vi "GCliWrite.vi"(8 "error in (no error)":errorcluster, 10 "Text to Write":string, 11 "CLI in":refnum<class "CLI.lvclass">) -> (0 "error out":errorcluster, 3 "CLI out":refnum<class "CLI.lvclass">)   [LabVIEW 2023, in "Reusables.lvlib"]
uses:
  Reusables.lvlib
  <vilib>/Wiresmith Technology/G CLI/CLI Class/CLI.lvclass
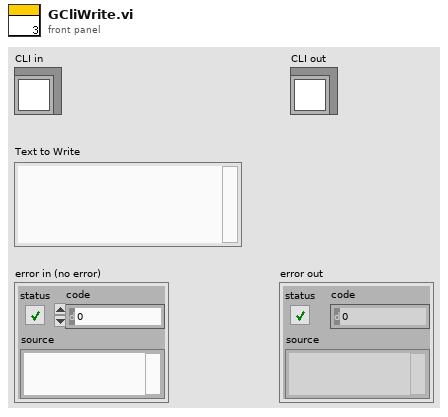
[diagram p1: front panel]
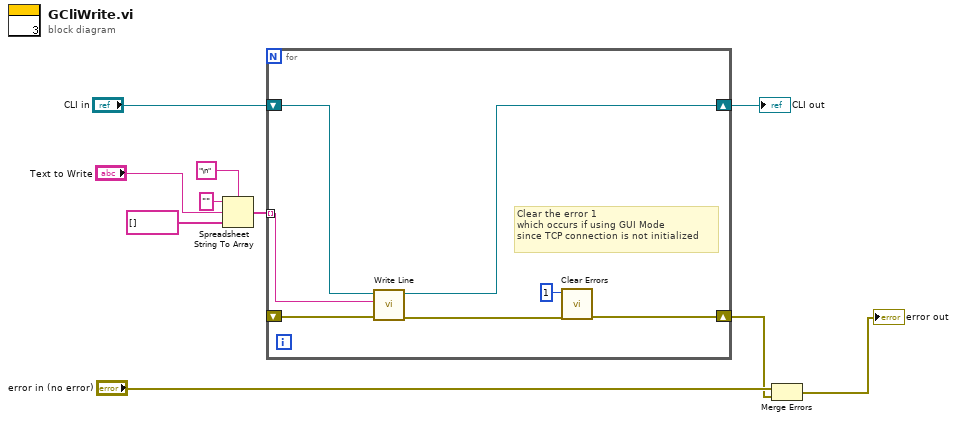
[diagram p0: block diagram]
diagram:
  n1 = Spreadsheet String To Array(delimiter (Tab)="\n", format string="", spreadsheet string="Text to Write", array type (2D Dbl)=string[] []) -> (array=w1:string[])
  n2 = for {
    shift-right: [w17] -> w10
    shift-left: "CLI in" -> [w16]
    tunnel: w1 -> [w12] mode=indexing
    shift-right: [w13] -> w7
    shift-left: _ -> [w11]
    # "Clear the error 1\nwhich occurs if using GUI Mode\nsince TCP connection is not initialized"
    n3 = call <vilib>:"Write Line.vi"("error in (no error)"=w11, "Text to Write"=w12, "CLI in"=w16) -> ("error out"=w15:errorcluster, "CLI out"=w17:refnum<class "CLI.lvclass">)  [unwired: 7 in]
    n4 = call <vilib>:"Clear Errors.vi"("error in (no error)"=w15, "specific error code to clear (0: all)"=1) -> ("error out"=w13:errorcluster)  [unwired: 4 in, 1 out]
  }
  "CLI out" <- w10
  n5 = Merge Errors("error in (no error)", w7) -> (→"error out":errorcluster)
